vi "Main.vi"() -> ()   [LabVIEW 2020]
uses:
  Global.vi
panel:
  in  "Il 1":bool
  in  "Il 2":bool
  in  "Il 3":bool
  in  "Il 4":bool
  out "Action4":bool
  out "Action3":bool
  out "Action2":bool
  out "Action1":bool
  in  "Machine in Cycle\nAuto":bool
  in  "STOP":bool
  in  "Initialize":bool
  in  "Tr 1":bool
  out "Cluster":cluster{string, "Interlock":bool, "Active":bool}
  out "Cluster 2":cluster{string, "Interlock":bool, "Active":bool}
  out "Cluster 3":cluster{string, "Interlock":bool, "Active":bool}
  out "Cluster 4":cluster{string, "Interlock":bool, "Active":bool}
  in  "Tr 2":bool
  in  "Tr 3":bool
  in  "Tr 4":bool
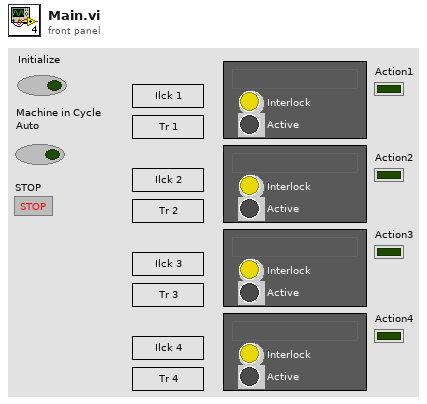
[diagram p1: front panel]
types:
  T1 = typedef "Data.ctl" = cluster{"Aktywny":bool, "Nazwa":string, "NrKroku":dbl, "Interlock":bool, "Akcja":bool, "Tranzycja":bool}
  T2 = cluster{"Array":T1[], "error":errorcluster, "Activate Next Step":bool, "NrKroku":dbl, "Auto":bool}
  T3 = cluster{T1[], "error":errorcluster, "Activate Next Step":bool, "NrKroku":dbl, "Auto":bool}
  T4 = cluster{string, "Interlock":bool, "Aktywny":bool}
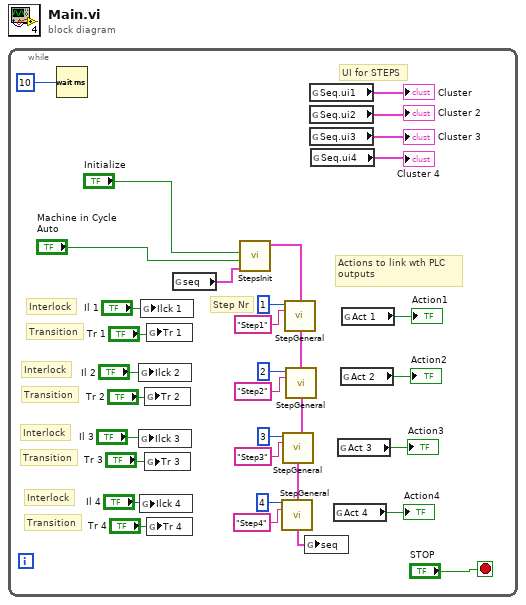
[diagram p0: block diagram]
diagram:
  n1 = while {
    stop <- "STOP" stop-if-true
    # "Actions to link wth PLC\noutputs"
    # "Transition"
    # "Interlock"
    # "Transition"
    # "Interlock"
    # "Transition"
    # "Interlock"
    # "Transition"
    # "UI for STEPS"
    # "Interlock"
    # "Step Nr"
    n2 = Wait (ms)(milliseconds to wait=u32 10 ("millisecond timer value")) -> ()  [unwired: 1 out]
    n3 = global write "Global.vi" "Ilck 2"("Il 2") -> ()
    n4 = global write "Global.vi" "Ilck 3"("Il 3") -> ()
    n5 = global write "Global.vi" "Ilck 4"("Il 4") -> ()
    n6 = global write "Global.vi" "Ilck 1"("Il 1") -> ()
    n7 = global write "Global.vi" "Tr 2"("Tr 2") -> ()
    n8 = global write "Global.vi" "Tr 3"("Tr 3") -> ()
    n9 = global write "Global.vi" "Tr 1"("Tr 1") -> ()
    n10 = global write "Global.vi" "Tr 4"("Tr 4") -> ()
    n11 = global read "Global.vi" "seq"() -> (w33:T2)
    n12 = call "StepsInit.vi"("Feedback"=w33, "Auto"="Machine in Cycle\nAuto", "Inicjalizuj"="Initialize") -> ("Cluster"=w15:T3)  [unwired: 8 in]
    n13 = call "StepGeneral.vi"("StepNr"=1, "seq in"=w15, "Nazwa"="Step1") -> ("seq out"=w7:T2)  [unwired: 12 in]
    n14 = call "StepGeneral.vi"("StepNr"=2, "seq in"=w7, "Nazwa"="Step2") -> ("seq out"=w6:T2)  [unwired: 12 in]
    n15 = call "StepGeneral.vi"("StepNr"=3, "seq in"=w6, "Nazwa"="Step3") -> ("seq out"=w5:T2)  [unwired: 12 in]
    n16 = call "StepGeneral.vi"("StepNr"=4, "seq in"=w5, "Nazwa"="Step4") -> ("seq out"=w8:T2)  [unwired: 12 in]
    n17 = global write "Global.vi" "seq"(w8) -> ()
    n18 = global read "Global.vi" "Seq.ui1"() -> (→"Cluster":T4)
    n19 = global read "Global.vi" "Seq.ui2"() -> (→"Cluster 2":T4)
    n20 = global read "Global.vi" "Seq.ui3"() -> (→"Cluster 3":T4)
    n21 = global read "Global.vi" "Seq.ui4"() -> (→"Cluster 4":T4)
    n22 = global read "Global.vi" "Act 4"() -> (→"Action4":bool)
    n23 = global read "Global.vi" "Act 3"() -> (→"Action3":bool)
    n24 = global read "Global.vi" "Act 2"() -> (→"Action2":bool)
    n25 = global read "Global.vi" "Act 1"() -> (→"Action1":bool)
  }
